vi "SetIntakeState.vi"(11 "inputState":enum16{"idle", "lower", "raise", "feed", "spit"}(ring)) -> ()   [LabVIEW 2017]
panel:
  # "input state enum"
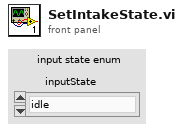
[diagram p1: front panel]
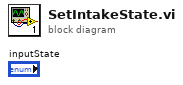
[diagram p0: block diagram]
diagram:
